vi "User Event.vi"() -> ()   [LabVIEW 2014]
doc: "This VI contains the Fire Event Boolean control that causes an LED to light when the user clicks the control. In addition, the block diagram contains a countdown that displays on the slider on the front panel. When the countdown reaches zero, a programmatic event fires that lights the LED."
panel:
  in  "Fire Event":bool
  in  "Stop":bool
  out "Loop 1 Stopped":bool
  out "Count Down to Event...":i32(slide) scale=0.0..100.0
  out "Event Count":i16
  out "Event Fired!":bool
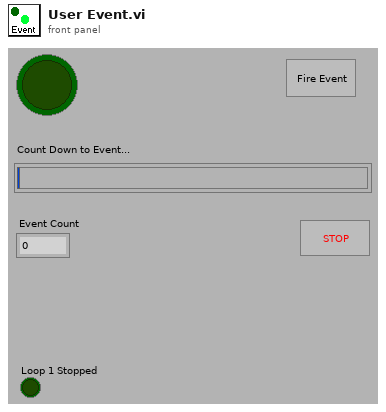
[diagram p1: front panel]
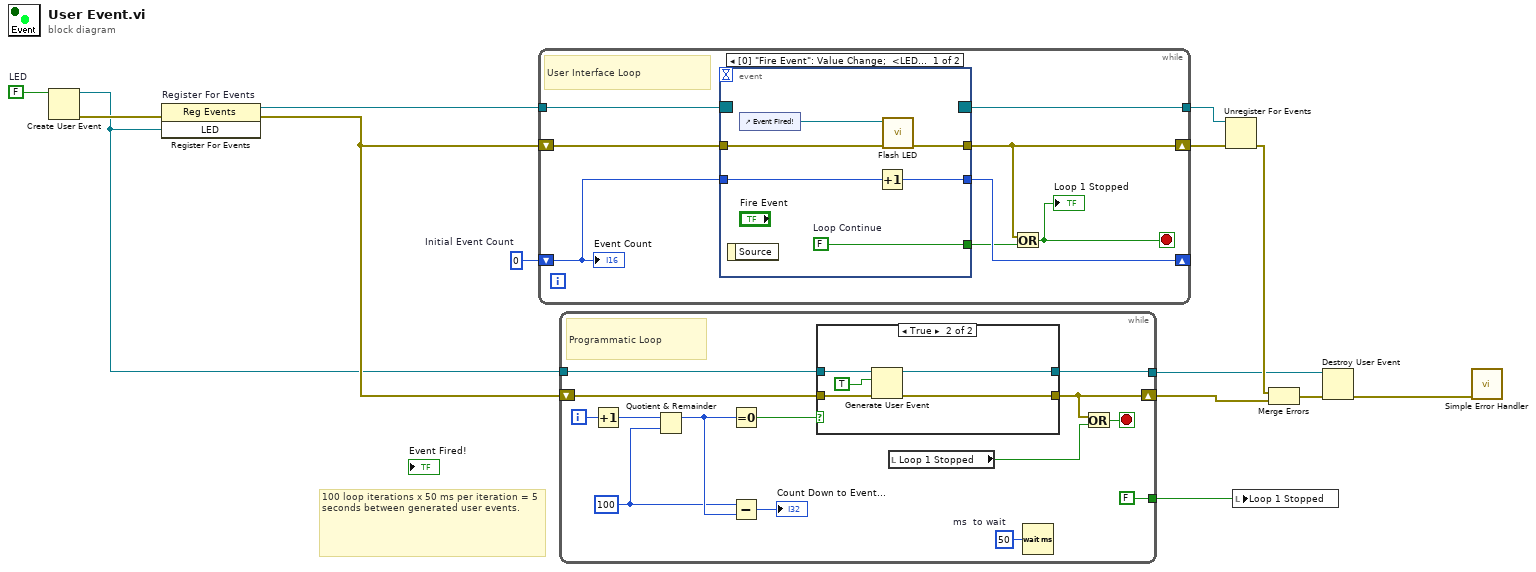
[diagram p0: block diagram]
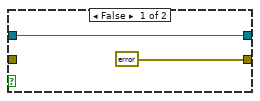
[diagram p2: hidden frame]
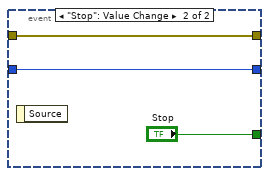
[diagram p3: hidden frame]
diagram:
  w11 = FALSE  # LED
  w14 = i16 0  # Initial Event Count
  # "100 loop iterations x 50 ms per iteration = 5 seconds between generated user events."
  n1 = Create User Event(user event datatype=w11) -> (user event=w8:refnum<user-event>, error out=w12:errorcluster)  [unwired: 1 in]
  n2 = register-events "Register For Events"(error in=w12, w8) -> (reference out=w10:refnum<event-registration>, error out=w9:errorcluster)  [unwired: 1 in]
  n3 = while {
    shift-right: [w18] -> _
    shift-left: w14 -> [w19]
    tunnel: w10 -> [w21]
    shift-right: [w15] -> w7
    shift-left: w9 -> [w20]
    tunnel: [w16] -> w6
    stop <- w22 stop-if-true
    # "User Interface Loop"
    n4 = event shown="[0] \"Fire Event\": Value Change;  <LED>: User Event" {
      selector: w21 -> [_ _]
      dyn-events: [_ _] -> w16
      timeout: _ -> [_ _]
      tunnel: w19 -> [w28 w30]
      tunnel: [w27 w30] -> w18
      tunnel: w20 -> [w26 w31]
      tunnel: [w25 w31] -> w15
      tunnel: [w24 "Stop"] -> w17
      event "Fire Event": Value Change; User Event {
        w24 = FALSE  # Loop Continue
        n5 = event-data() -> ()  [unwired: 1 in, 1 out]
        n6 = control-ref of="Event Fired!"() -> (w23:refnum<vi>)
        n7 = Increment(x=w28) -> (x+1=w27:i16)
        n8 = call "Flash LED.vi"("error in"=w26, "Bool Refnum"=w23) -> ("error out"=w25:errorcluster)  [unwired: 5 in]
      }
      event "Stop": Value Change {
        n9 = event-data() -> ()  [unwired: 1 in, 1 out]
      }
    }
    n10 = Or(x=w15, y=w17) -> (x .or. y?=w22:bool)
    "Loop 1 Stopped" <- w22
    "Event Count" <- w19
  }
  n11 = while {
    shift-right: [w32] -> w5
    shift-left: w9 -> [w38]
    tunnel: [FALSE] -> w13
    tunnel: w8 -> [w34]
    tunnel: [w33] -> w2
    i -> [w41]
    stop <- w36 stop-if-true
    w39 = u32 50  # ms  to wait
    w43 = 100 ("y")
    # "Programmatic Loop"
    n12 = Increment(x=w41) -> (x+1=w42:i32)
    n13 = Quotient & Remainder(x=w42, y=w43) -> (x-y*floor(x/y)=w44:i32)  [unwired: 1 out]
    n14 = Equal To 0?(x=w44) -> (x = 0?=w40:bool)
    n15 = Subtract(x=w43, y=w44) -> (x-y=→"Count Down to Event...":i32)
    n16 = case shown="True" w40 {
      tunnel: [errorcluster {"status"=FALSE, "code"=0, "source"=""} ("error out") w51] -> w32
      tunnel: w38 -> [_ w52]
      tunnel: w34 -> [w47 w49]
      tunnel: [w47 w48] -> w33
      frame False {
      }
      frame True {
        n17 = Generate User Event(user event=w49, event data cluster=TRUE, error in=w52) -> (user event out=w48:refnum<user-event>, error out=w51:errorcluster)  [unwired: 1 in]
      }
    }
    n18 = local read "Loop 1 Stopped"() -> (w37:bool)
    n19 = Wait (ms)(milliseconds to wait=w39) -> ()  [unwired: 1 out]
    n20 = Or(x=w32, y=w37) -> (x .or. y?=w36:bool)
  }
  n21 = Unregister For Events(event registration refnum=w6, error in=w7) -> (error out=w4:errorcluster)
  n22 = local write "Loop 1 Stopped"(w13) -> ()
  n23 = Merge Errors(w4, w5) -> (w3:errorcluster)
  n24 = Destroy User Event(user event=w2, error in=w3) -> (error out=w1:errorcluster)
  n25 = call <vilib>:"Simple Error Handler.vi"("error in (no error)"=w1) -> ()  [unwired: 4 in, 5 out]
